vi "Initialize Attributes Core.vi"(8 "error in (no error)":errorcluster, 10 "Attribute Data":variant, 11 "BNT_DSCXtGraph in":refnum<class "BNT_DSCXtGraph.lvclass">) -> (0 "error out":errorcluster, 2 "MandatoryParameters":cluster{"Parameter":string, "found?":bool}[](array[cluster]), 3 "BNT_DSCXtGraph out":refnum<class "BNT_DSCXtGraph.lvclass">)   [LabVIEW 2018, in "BNT_DSCXtGraph.lvlib" / "BNT_DSCXtGraph.lvclass"]
doc: "Initialize object attribute.\n\nUnique resources should be allocated elsewhere!"
uses:
  BNT_DSCXtGraph.lvclass
  BNT_DSCXtGraph.lvclass/BNT_DSCXtGraph.ctl
  CSPP_Core/Actors/CSPP_GUIActor/CSPP_GUIActor.lvclass
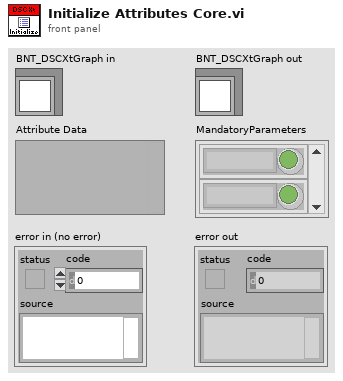
[diagram p1: front panel]
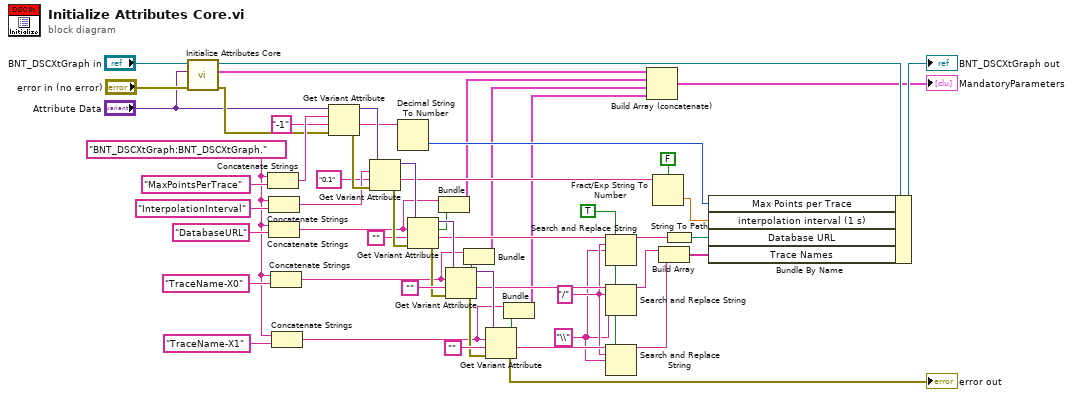
[diagram p0: block diagram]
diagram:
  w18 = TRUE ("replace all? (F)")
  w16 = "\\" ("replace string (\"\")")
  w17 = "/" ("search string")
  w44 = "BNT_DSCXtGraph:BNT_DSCXtGraph."
  n1 = call-parent "Initialize Attributes Core.vi"("error in (no error)"="error in (no error)", "Attribute Data"="Attribute Data", "CSPP_GUIActor in"="BNT_DSCXtGraph in") -> ("error out"=w50:errorcluster, "MandatoryParameters"=w51:cluster{"Parameter":string, "found?":bool}[], "CSPP_GUIActor out"=w25:refnum<class "BNT_DSCXtGraph.lvclass">)  [unwired: 6 in]
  n2 = Concatenate Strings(w44, "MaxPointsPerTrace" ("string")) -> (w55:string)
  n3 = Concatenate Strings(w44, "InterpolationInterval" ("string")) -> (w52:string)
  n4 = Concatenate Strings(w44, "DatabaseURL" ("string")) -> (w9:string)
  n5 = Concatenate Strings(w44, "TraceName-X0" ("string")) -> (w6:string)
  n6 = Concatenate Strings(w44, "TraceName-X1" ("string")) -> (w3:string)
  n7 = Get Variant Attribute(Variant="Attribute Data", name=w55, default value (empty Variant)="-1" ("string"), error in=w50) -> (duplicate Variant=w54:variant, value=w30:string, error out=w53:errorcluster)  [unwired: 1 out]
  n8 = Get Variant Attribute(Variant=w54, name=w52, default value (empty Variant)="0.1" ("string"), error in=w53) -> (duplicate Variant=w41:variant, value=w28:string, error out=w40:errorcluster)  [unwired: 1 out]
  n9 = Decimal String To Number(string=w30) -> (number=w29:i32)  [unwired: 2 in, 1 out]
  n10 = Get Variant Attribute(Variant=w41, name=w9, default value (empty Variant)="", error in=w40) -> (duplicate Variant=w37:variant, found=w8:bool, value=w19:string, error out=w36:errorcluster)
  n11 = Bundle(w9, w8) -> (w7:cluster{string, bool})  [unwired: 1 in]
  n12 = Get Variant Attribute(Variant=w37, name=w6, default value (empty Variant)="", error in=w36) -> (duplicate Variant=w33:variant, found=w5:bool, value=w24:string, error out=w34:errorcluster)
  n13 = Bundle(w6, w5) -> (w4:cluster{string, bool})  [unwired: 1 in]
  n14 = Get Variant Attribute(Variant=w33, name=w3, default value (empty Variant)="", error in=w34) -> (found=w2:bool, value=w22:string, error out=→"error out":errorcluster)  [unwired: 1 out]
  n15 = Bundle(w3, w2) -> (w1:cluster{string, bool})  [unwired: 1 in]
  n16 = Search and Replace String(replace all?=w18, input string=w19, search string=w17, replace string=w16) -> (result string=w20:string)  [unwired: 4 in, 3 out]
  n17 = Search and Replace String(replace all?=w18, input string=w24, search string=w17, replace string=w16) -> (result string=w23:string)  [unwired: 4 in, 3 out]
  n18 = Search and Replace String(replace all?=w18, input string=w22, search string=w17, replace string=w16) -> (result string=w21:string)  [unwired: 4 in, 3 out]
  n19 = Build Array (concatenate)(w51, w7, w4, w1) -> (→"MandatoryParameters":cluster{"Parameter":string, "found?":bool}[])
  n20 = Fract/Exp String To Number(use system decimal point (T)=FALSE, string=w28) -> (number=w27:dbl)  [unwired: 2 in, 1 out]
  n21 = Build Array(w23, w21) -> (w31:string[])
  n22 = String To Path(string=w20) -> (path=w32:path)
  n23 = Bundle By Name(cluster=w25, "Max Points per Trace"=w29, "interpolation interval (1 s)"=w27, "Database URL"=w32, "Trace Names"=w31) -> (→"BNT_DSCXtGraph out":refnum<class "BNT_DSCXtGraph.lvclass">)
